vi "Read From DRAM Ref.vi"(8 "error in (no error)":errorcluster, 11 "K7 DRAM FIFO in":refnum<class "K7 DRAM FIFO.lvclass">) -> (0 "error out":errorcluster, 2 "From DRAM":refnum<k21>, 3 "K7 DRAM FIFO out":refnum<class "K7 DRAM FIFO.lvclass">)   [LabVIEW 2014, in "K7 DRAM FIFO.lvclass"]
uses:
  K7 DRAM FIFO.lvclass
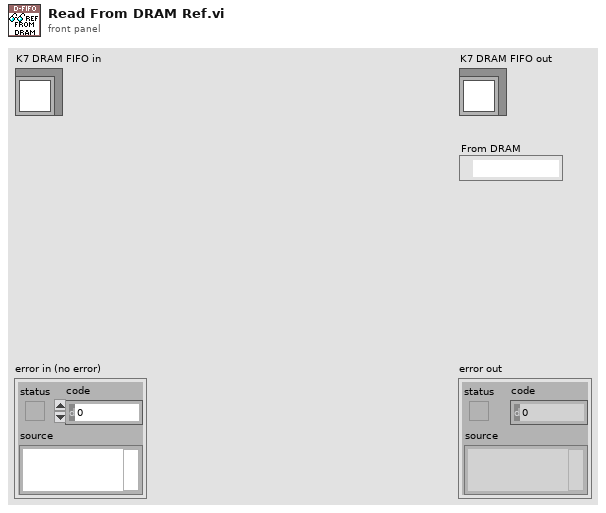
[diagram p1: front panel]
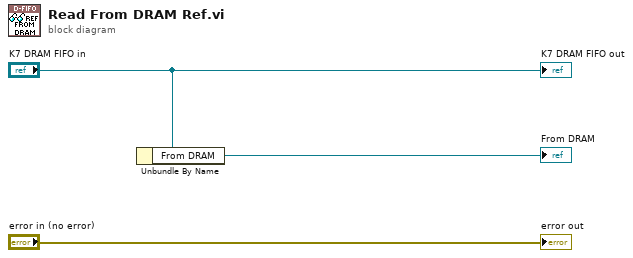
[diagram p0: block diagram]
diagram:
  n1 = Unbundle By Name("K7 DRAM FIFO in") -> ("From DRAM"=→"From DRAM":refnum<k21>)
  "error out" <- "error in (no error)"
  "K7 DRAM FIFO out" <- "K7 DRAM FIFO in"
